vi "RT1.vi"() -> ()   [LabVIEW 2017]
doc: "This example shows how to configure the instrument's output voltage level, over current protection, and over voltage protection. The actual voltage level and actual current level are returned as well as whether over voltage protection (OVP) or over current protection (OCP) has been tripped."
uses:
  <vilib>/Utility/file.llb/Write Delimited Spreadsheet (string).vi
  <instrlib>/Lake Shore 336/Public/Data/Sensor Data (Single Reading).vi
  <vilib>/Utility/file.llb/Write Delimited Spreadsheet (DBL).vi
  <instrlib>/Agilent B2900 Series/Agilent B2900 Series.lvlib
  <instrlib>/Lake Shore 336/Lake Shore 336.lvlib
panel:
  in  "?":enum32{"Controll", "Data Visualisation"}(tab)
  out "Measured Resistance (V/I)":dbl format="%_6g"
  in  "SMU address":refnum<visa-resource-name>
  out "Measured Voltage (V)":dbl format="%_6g"
  out "Measured Current (A)":dbl format="%_6g"
  in  "Stop":bool
  in  "Enable Output Protection (T: Enable)":bool=TRUE
  in  "Source Range (A)":dbl=2.0
  in  "Source current (A)":dbl
  in  "Compliance Voltage (2 V)":dbl=2.0 format="%#_13g"
  in  "Temperature controller address":refnum<visa-resource-name>
  in  "Output's Control Loop (1:1)":u16(ring)=1 items=["1"=1, "2"=2]
  in  "Configure Control Parameters (0: Configure)":u16(ring) items=["Configure", "Don't Configure"]
  in  "Heater Range (Low)":u16(ring) items=["Off", "Low (On)", "Medium", "High"]
  in  "Manual Output (0.00 %)":dbl format="%.2f"
  in  "Rate (D) (0.0 %)":dbl format="%.1f"
  in  "Reset (I) (20.0)":dbl=20.0 format="%.1f"
  in  "Gain (P) (50.0)":dbl=50.0 format="%.1f"
  in  "Max Current (if specified by user)":dbl=2.0 format="%.3f"
  in  "Max Current (0:User Specified)":u16(ring) items=["User Specified", "0.707 A", "1.0 A", "1.141 A", "2.0 A"]
  in  "Controll mode  (0:Off)":u16(ring) items=["Off", "Closed Loop PID", "Zone", "Open Loop"]
  in  "Input (0:None)":u16(ring) items=["None", "A", "B", "C", "D"]
  in  "Enable Setpoint (F:Off)":bool
  in  "Setpoint (0.00000)":dbl format="%.5f"
  in  "Input 1 (0:A)":u16(ring) items=["A", "B", "C", "D"]
  out "Sensor Data 1":dbl format="%.4f"
  in  "Setpoint Ramping \nEnable (F: Off)":bool
  in  "Ramp Rate K/min (0.0)":dbl format="%.1f"
  in  "Input 2":u16(ring) items=["A", "B", "C", "D"]
  out "Sensor Data 2":dbl format="%.4f"
  in  "centiseconds to wait (0.1 seconds)":u64=60000
  in  "Save data at":path
  # "Resistance vs Temperature Measurement"
  # "Heater Parameters"
  # "Compliance Protection"
  # "Sensor Data"
  # "Setpoint"
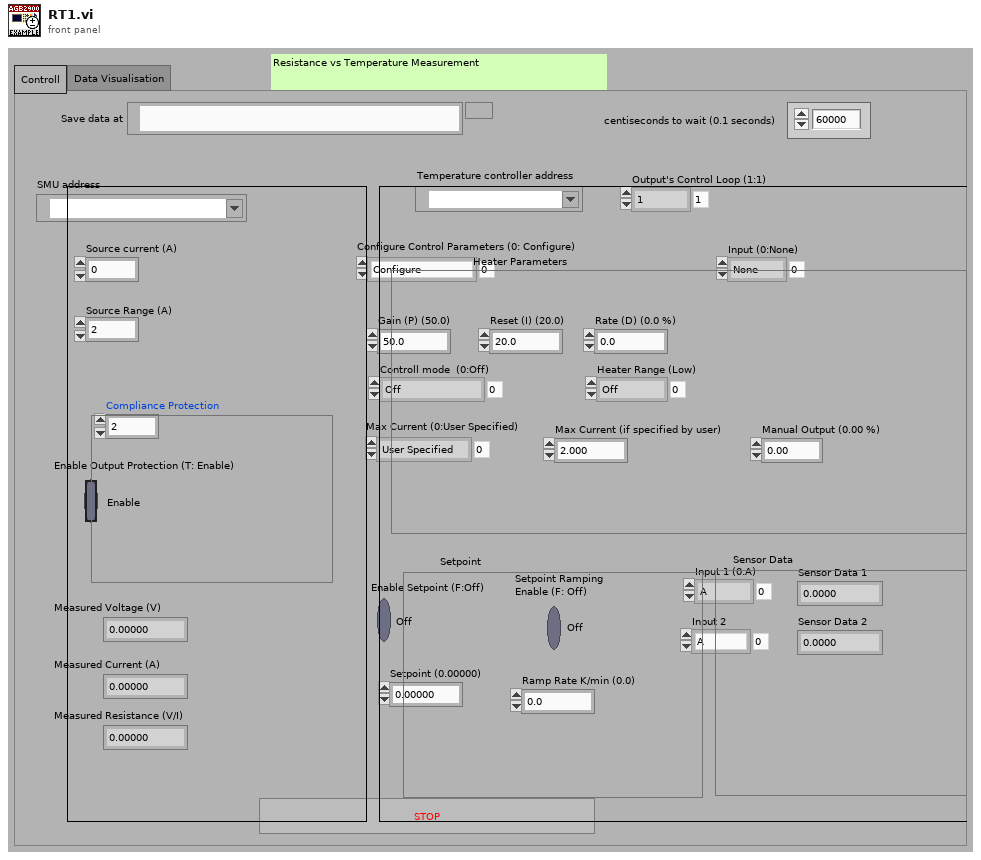
[diagram p1: front panel]
types:
  T1 = cluster{"Baud Rate":u32, "Parity":u16, "Data Bits":u16, "Stop Bits":u16, "Flow Control":u16}
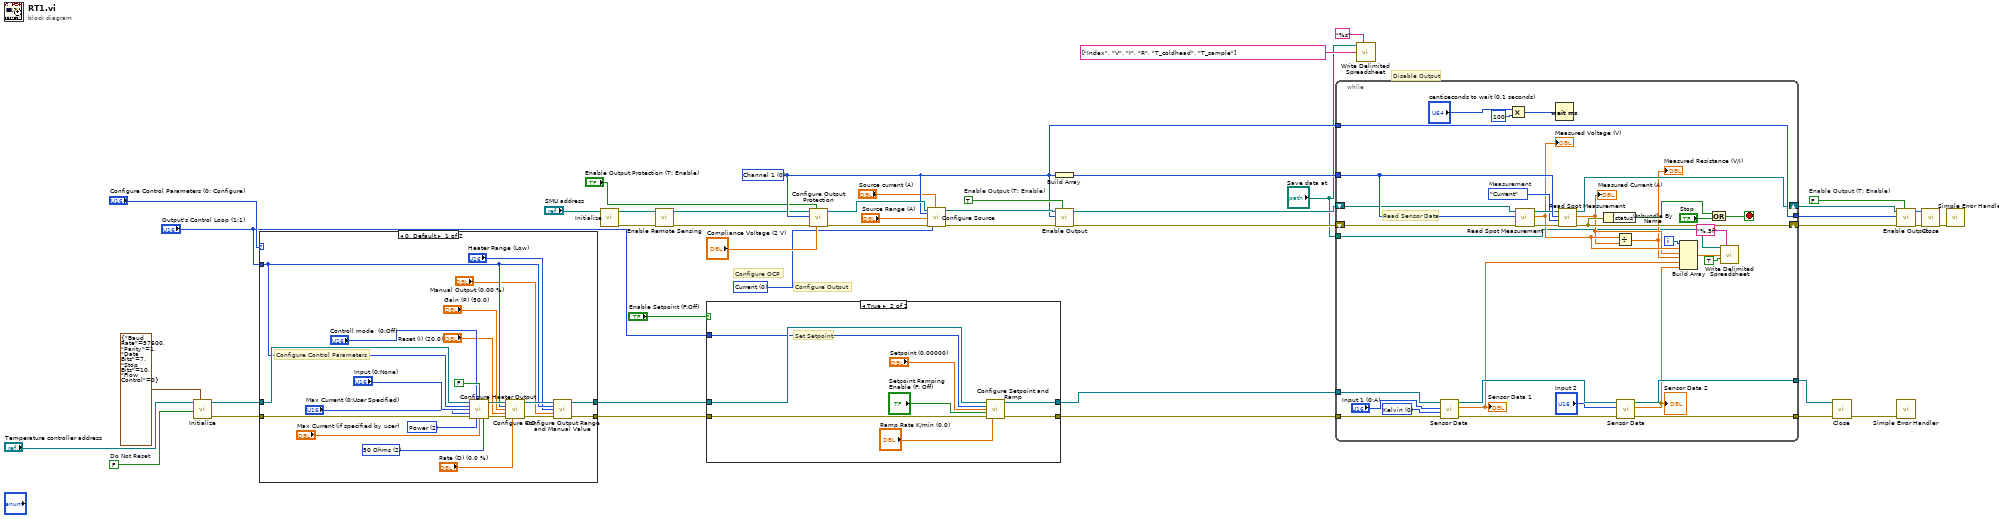
[diagram p0: block diagram]
diagram:
  w10 = FALSE  # Do Not Reset
  w28 = 0 items=["Channel 1", "Channel 2"] ("Channel (0: Channel 1)")
  w23 = 0 items=["Current", "Voltage"] ("Source Mode (1: Voltage)")
  w35 = FALSE  # Enable Output (T: Enable)
  w34 = TRUE  # Enable Output (T: Enable)
  # "Disable Output"
  # "Configure Output"
  # "Configure OCP"
  n1 = call <instrlib>:"Initialize.vi"("Serial Configuration"=T1 {"Baud Rate"=57600, "Parity"=1, "Data Bits"=7, "Stop Bits"=10, "Flow Control"=0}, "Reset (True)"=w10, "VISA resource name"="Temperature controller address") -> ("error out"=w17:errorcluster, "VISA resource name out"=w18:refnum<visa-resource-name>)  [unwired: 7 in]
  n2 = case shown="0, Default" "Configure Control Parameters (0: Configure)" {
    tunnel: "Output's Control Loop (1:1)" -> [w50 _]
    tunnel: w18 -> [w65 w67]
    tunnel: w17 -> [w64 w66]
    tunnel: [w59 w66] -> w11
    tunnel: [w58 w67] -> w12
    frame 0, Default {
      w51 = u16 2 items=["25 Ohms"=1, "50 Ohms"=2] ("Heater Resistance (1:25 Ohms)")
      w53 = u16 2 items=["Current"=1, "Power"=2] ("Heater Out Display (1:Current)")
      # "Configure Control Parameters"
      n3 = call <instrlib>:"Configure Heater Output.vi"("VISA resource name"=w65, "Mode (0:Off)"="Controll mode  (0:Off)", "Power Up Enable (F: Off)"=FALSE, "Heater Output (1:1)"=w50, "Input (0:None)"="Input (0:None)", "Max Current (0:User Specified)"="Max Current (0:User Specified)", "error in (no error)"=w64, "Heater Out Display (1:Current)"=w53, "Max User Current (2.000)"="Max Current (if specified by user)", "Heater Resistance (1:25 Ohms)"=w51) -> ("VISA resource name out"=w62:refnum<visa-resource-name>, "error out"=w63:errorcluster)  [unwired: 4 in]
      n4 = call <instrlib>:"Configure PID.vi"("VISA resource name"=w62, "Output's Control Loop (1:1)"=w50, "Gain (P) (50.0)"="Gain (P) (50.0)", "Reset (I) (20.0)"="Reset (I) (20.0)", "error in (no error)"=w63, "Rate (D) (0.0 %)"="Rate (D) (0.0 %)") -> ("VISA resource name out"=w61:refnum<visa-resource-name>, "error out"=w60:errorcluster)  [unwired: 8 in]
      n5 = call <instrlib>:"Configure Output Range and Manual Value.vi"("VISA resource name"=w61, "Output (1:1)"=w50, "Range (0:Off)"="Heater Range (Low)", "Manual Output (0.00 %)"="Manual Output (0.00 %)", "error in (no error)"=w60) -> ("VISA resource name out"=w58:refnum<visa-resource-name>, "error out"=w59:errorcluster)  [unwired: 9 in]
    }
    frame 1 {
      # "Do Not Configure Control Parameters"
    }
  }
  n6 = call <instrlib>:"Initialize.vi"("VISA resource name"="SMU address") -> ("error out"=w20:errorcluster, "VISA resource name out"=w22:refnum<visa-resource-name>)  [unwired: 9 in]
  n7 = call <instrlib>:"Enable Remote Sensing.vi"("error in (no error)"=w20, "VISA resource name"=w22) -> ("error out"=w19:errorcluster, "VISA resource name out"=w21:refnum<visa-resource-name>)  [unwired: 8 in]
  n8 = case shown="True" "Enable Setpoint (F:Off)" {
    tunnel: "Output's Control Loop (1:1)" -> [_ w75]
    tunnel: w12 -> [w69 w76]
    tunnel: w11 -> [w68 w77]
    tunnel: [w68 w72] -> w7
    tunnel: [w69 w73] -> w6
    frame False {
      # "Do Not Set Setpoint"
    }
    frame True {
      # "Set Setpoint"
      n9 = call <instrlib>:"Configure Setpoint and Ramp.vi"("VISA resource name"=w76, "Output's Control Loop (1:1)"=w75, "Setpoint (0.00000)"="Setpoint (0.00000)", "Setpoint Ramping \nEnable (F: Off)"="Setpoint Ramping \nEnable (F: Off)", "error in (no error)"=w77, "Ramp Rate (0.0)"="Ramp Rate K/min (0.0)") -> ("VISA resource name out"=w73:refnum<visa-resource-name>, "error out"=w72:errorcluster)  [unwired: 8 in]
    }
  }
  n10 = call <instrlib>:"Configure Output Protection.vi"("Compliance Voltage (2 V)"="Compliance Voltage (2 V)", "Enable Output Protection (T: Enable)"="Enable Output Protection (T: Enable)", "error in (no error)"=w19, "Channel (0: Channel 1)"=w28, "VISA resource name"=w21) -> ("error out"=w31:errorcluster, "VISA resource name out"=w32:refnum<visa-resource-name>)  [unwired: 5 in]
  n11 = call <instrlib>:"Configure Source.vi"("VISA resource name"=w32, "Channel (0: Channel 1)"=w28, "Source Range (2)"="Source Range (A)", "error in (no error)"=w31, "Source Mode (1: Voltage)"=w23, "Output Level (0)"="Source current (A)") -> ("VISA resource name out"=w30:refnum<visa-resource-name>, "error out"=w29:errorcluster)  [unwired: 12 in]
  n12 = Build Array(w28) -> (w33:i32[])
  n13 = call <instrlib>:"Enable Output.vi"("Enable Output (T: Enable)"=w34, "error in (no error)"=w29, "Channel (0: Channel 1)"=w28, "VISA resource name"=w30) -> ("error out"=w41:errorcluster, "VISA resource name out"=w42:refnum<visa-resource-name>)  [unwired: 5 in, 1 out]
  n14 = while {
    tunnel: w28 -> [w111]
    tunnel: [w111] -> w40
    shift-right: [w102] -> w39
    shift-left: w41 -> [w101]
    tunnel: w33 -> [w109]
    shift-right: [w110] -> w36
    shift-left: w42 -> [w100]
    tunnel: w7 -> [w99]
    tunnel: w6 -> [w98]
    tunnel: [w94] -> w5
    tunnel: [w96] -> w4
    tunnel: "Save data at" -> [w80]
    i -> [w86]
    stop <- w106 stop-if-true
    w92 = u16 0 items=["Kelvin", "Celsius", "Sensor Units"] ("Data Source (0:Kelvin)")
    w103 = enum16{"Voltage", "Current", "Resistance"}."Current"  # Measurement
    # "Read Sensor Data"
    n15 = call-poly <instrlib>:"Sensor Data.vi"("error in (no error)"=w99, "Data Source (0:Kelvin)"=w92, "Input (0:A)"="Input 1 (0:A)", "VISA resource name"=w98) -> ("error out"=w95:errorcluster, "Sensor Data"=w82:dbl, "VISA resource name out"=w97:refnum<visa-resource-name>)  [unwired: 5 in]
    "Sensor Data 1" <- w82
    n16 = Multiply(x="centiseconds to wait (0.1 seconds)", y=u32 100) -> (x*y=w91:u64)
    n17 = call <instrlib>:"Read Spot Measurement.vi"("error in (no error)"=w101, "Channel List ({Channel1})"=w109, "VISA resource name"=w100) -> ("error out"=w105:errorcluster, "Measurement Result"=w85:dbl, "VISA resource name out"=w104:refnum<visa-resource-name>)  [unwired: 6 in]
    "Measured Voltage (V)" <- w85
    n18 = Wait (ms)(milliseconds to wait=w91) -> ()  [unwired: 1 out]
    n19 = call <instrlib>:"Read Spot Measurement.vi"("error in (no error)"=w105, "Measurement Mode (0:Voltage)"=w103, "Channel List ({Channel1})"=w109, "VISA resource name"=w104) -> ("error out"=w102:errorcluster, "Measurement Result"=w84:dbl, "VISA resource name out"=w110:refnum<visa-resource-name>)  [unwired: 5 in]
    "Measured Current (A)" <- w84
    n20 = Unbundle By Name(w102) -> ("status"=w108:bool)
    n21 = Divide(x=w85, y=w84) -> (x/y=w83:dbl)
    "Measured Resistance (V/I)" <- w83
    n22 = call-poly <instrlib>:"Sensor Data.vi"("error in (no error)"=w95, "Input (0:A)"="Input 2", "VISA resource name"=w97) -> ("error out"=w94:errorcluster, "Sensor Data"=w81:dbl, "VISA resource name out"=w96:refnum<visa-resource-name>)  [unwired: 6 in]
    "Sensor Data 2" <- w81
    n23 = Build Array(w86, w85, w84, w83, w82, w81) -> (w87:dbl[])
    n24 = Compound Arithmetic op=OR(w108, "Stop") -> (w106:bool)
    n25 = call-poly <vilib>:"Write Delimited Spreadsheet.vi"("file path (dialog if empty)"=w80, "format (%.3f)"="%.5f", "1D data"=w87, "append to file? (new file:F)"=TRUE) -> ()  [unwired: 10 in, 2 out]
  }
  n26 = call-poly <vilib>:"Write Delimited Spreadsheet.vi"("file path (dialog if empty)"="Save data at", "format (%s)"="%s" ("format (%.3f)"), "1D data"=string[] ["Index", "V", "I", "R", "T_coldhead", "T_sample"]) -> ()  [unwired: 11 in, 2 out]
  n27 = call <instrlib>:"Close.vi"("error in (no error)"=w5, "VISA resource name"=w4) -> ("error out"=w13:errorcluster)  [unwired: 9 in]
  n28 = call <instrlib>:"Enable Output.vi"("Enable Output (T: Enable)"=w35, "error in (no error)"=w39, "Channel (0: Channel 1)"=w40, "VISA resource name"=w36) -> ("error out"=w37:errorcluster, "VISA resource name out"=w38:refnum<visa-resource-name>)  [unwired: 5 in, 1 out]
  n29 = call <vilib>:"Simple Error Handler.vi"("error in (no error)"=w13) -> ()  [unwired: 4 in, 5 out]
  n30 = call <instrlib>:"Close.vi"("error in (no error)"=w37, "VISA resource name"=w38) -> ("error out"=w43:errorcluster)  [unwired: 9 in]
  n31 = call <vilib>:"Simple Error Handler.vi"("error in (no error)"=w43) -> ()  [unwired: 4 in, 5 out]
